vi "RW_LiveVIew.vi"(9 "Task":T2(ring), 11 "Plots":refnum<vi>[](array[refnum])) -> ()   [LabVIEW 2022 SP3]
uses:
  <vilib>/Utility/miscctls.llb/LVRangeTypeDef.ctl
panel:
  out "Data":T1[][](array[typedef])
  out "Pref Path":path
  out "File Out":string
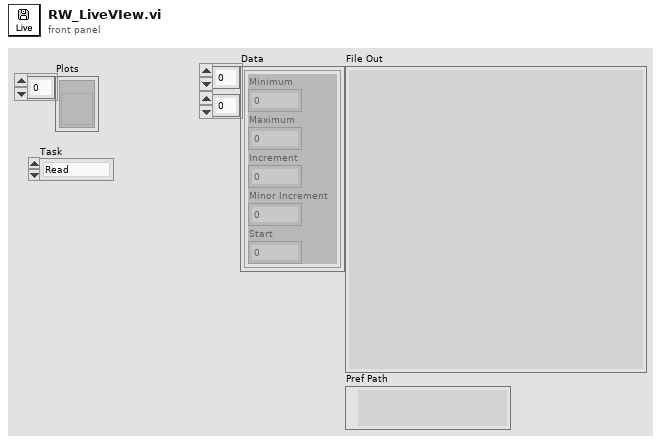
[diagram p1: front panel]
types:
  T1 = typedef "LVRangeTypeDef.ctl" = cluster{"Minimum":dbl, "Maximum":dbl, "Increment":dbl, "Minor Increment":dbl, "Start":dbl}
  T2 = enum16{"Read", "Write", "Init", "remember", "retrieve"}
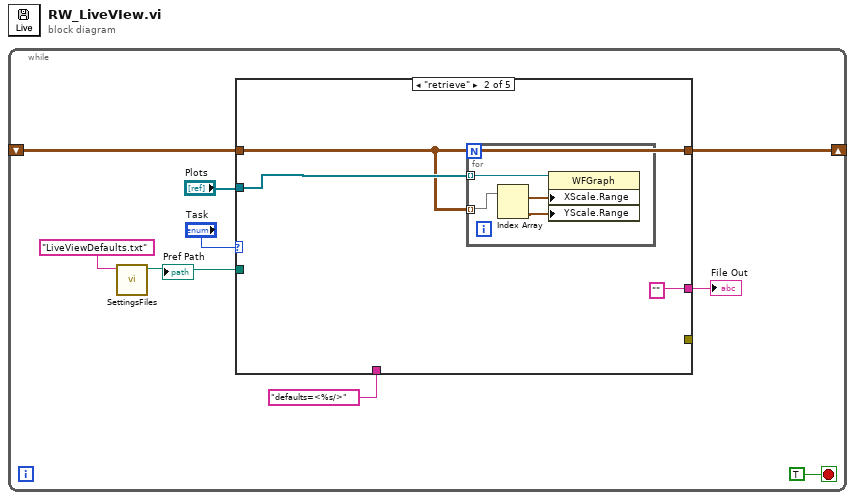
[diagram p0: block diagram]
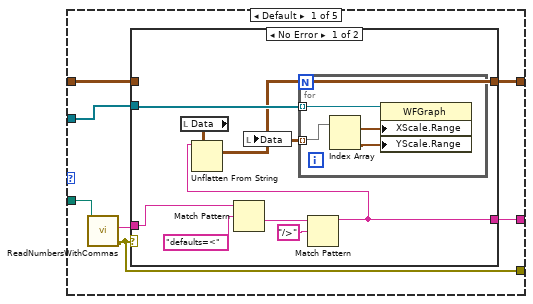
[diagram p2: hidden frame]
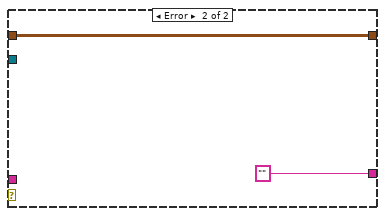
[diagram p3: hidden frame]
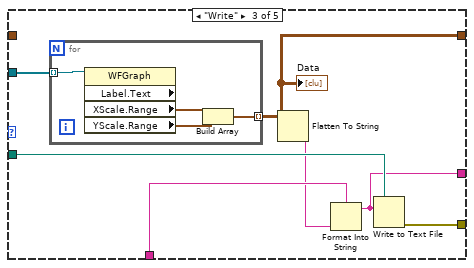
[diagram p4: hidden frame]
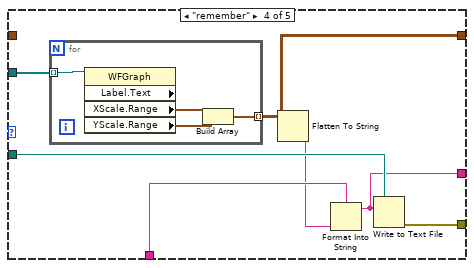
[diagram p5: hidden frame]
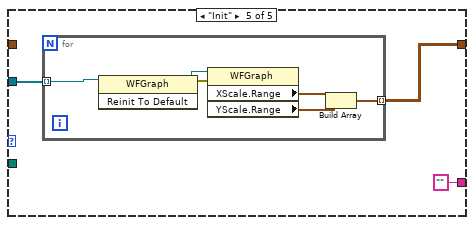
[diagram p6: hidden frame]
diagram:
  n1 = while {
    shift-right: [w3] -> _
    shift-left: _ -> [w2]
    stop <- TRUE stop-if-true
    n2 = call "SettingsFiles.vi"("settings file name"="LiveViewDefaults.txt" ("name or relative path")) -> ("file path"=w4:path)  [unwired: 9 in, 1 out]
    "Pref Path" <- w4
    n3 = case shown="\"retrieve\"" "Task" {
      tunnel: w4 -> [w16 _ w44 w55 _]
      tunnel: [w14 _ w43 w54 _] -> _
      tunnel: [w13 "" ("Notes") w39 w50 "" ("Notes")] -> w9
      tunnel: "defaults=<%s/>" ("format string") -> [_ _ w42 w53 _]
      tunnel: "Plots" -> [w12 w33 w41 w52 w62]
      tunnel: [w11 w32 w38 w49 w60] -> w3
      tunnel: w2 -> [w10 w32 _ _ _]
      frame Default {
        n4 = call "ReadNumbersWithCommas.vi"("file (use dialog)"=w16) -> ("error out"=w14:errorcluster, "text"=w15:string)  [unwired: 7 in, 2 out]
        n5 = case shown="No Error" w14 {
          tunnel: [w18 "" ("Notes")] -> w13
          tunnel: w15 -> [w24 _]
          tunnel: w12 -> [w19 _]
          tunnel: [w17 w29] -> w11
          tunnel: w10 -> [_ w29]
          frame No Error {
            n6 = local read "Data"() -> (w20:T1[][])
            n7 = Match Pattern(string=w24, regular expression="defaults=<" ("format string")) -> (after substring=w23:string)  [unwired: 1 in, 3 out]
            n8 = Match Pattern(string=w23, regular expression="/>" ("format string")) -> (before substring=w18:string)  [unwired: 1 in, 3 out]
            n9 = Unflatten From String(type=w20, binary string=w18) -> (value=w17:T1[][])  [unwired: 3 in, 2 out]
            n10 = local write "Data"(w17) -> ()
            n11 = for {
              tunnel: w19 -> [w28] mode=indexing
              tunnel: w17 -> [w27] mode=indexing
              n12 = Index Array(array=w27) -> (element #1=w26:T1, element #2=w25:T1)  [unwired: 2 in]
              n13 = property on="Property Node" class="WFGraph"(reference=w28, "XScale.Range"=w26, "YScale.Range"=w25) -> ()  [unwired: 1 in, 2 out]
            }
          }
          frame Error {
          }
        }
      }
      frame "retrieve" {
        n14 = for {
          tunnel: w33 -> [w37] mode=indexing
          tunnel: w32 -> [w36] mode=indexing
          n15 = Index Array(array=w36) -> (element #1=w35:T1, element #2=w34:T1)  [unwired: 2 in]
          n16 = property on="Property Node" class="WFGraph"(reference=w37, "XScale.Range"=w35, "YScale.Range"=w34) -> ()  [unwired: 1 in, 2 out]
        }
      }
      frame "Write" {
        n17 = for {
          tunnel: w41 -> [w48] mode=indexing
          tunnel: [w45] -> w38 mode=indexing
          n18 = property on="Property Node" class="WFGraph" props=["Label", "Text", "XScale", "Range", "YScale", "Range"](reference=w48) -> ("XScale.Range"=w47:T1, "YScale.Range"=w46:T1)  [unwired: 1 in, 3 out]
          n19 = Build Array(w47, w46) -> (w45:T1[])
        }
        "Data" <- w38
        n20 = Flatten To String(anything=w38) -> (data string=w40:string)  [unwired: 3 in, 2 out]
        n21 = Format Into String(format string=w42, w40) -> (resulting string=w39:string)  [unwired: 2 in, 1 out]
        n22 = Write to Text File(file (use dialog)=w44, text=w39) -> (error out=w43:errorcluster)  [unwired: 2 in, 2 out]
      }
      frame "remember" {
        n23 = for {
          tunnel: w52 -> [w59] mode=indexing
          tunnel: [w56] -> w49 mode=indexing
          n24 = property on="Property Node" class="WFGraph" props=["Label", "Text", "XScale", "Range", "YScale", "Range"](reference=w59) -> ("XScale.Range"=w58:T1, "YScale.Range"=w57:T1)  [unwired: 1 in, 3 out]
          n25 = Build Array(w58, w57) -> (w56:T1[])
        }
        n26 = Flatten To String(anything=w49) -> (data string=w51:string)  [unwired: 3 in, 2 out]
        n27 = Format Into String(format string=w53, w51) -> (resulting string=w50:string)  [unwired: 2 in, 1 out]
        n28 = Write to Text File(file (use dialog)=w55, text=w50) -> (error out=w54:errorcluster)  [unwired: 2 in, 2 out]
      }
      frame "Init" {
        n29 = for {
          tunnel: w62 -> [w68] mode=indexing
          tunnel: [w65] -> w60 mode=indexing
          n30 = invoke on="Invoke Node" class="WFGraph" method="Reinit To Default"(reference=w68) -> (reference out=w64:refnum<vi>, error out=w63:errorcluster)  [unwired: 2 in, 1 out]
          n31 = property on="Property Node" class="WFGraph"(reference=w64, error in=w63) -> ("XScale.Range"=w67:T1, "YScale.Range"=w66:T1)  [unwired: 2 out]
          n32 = Build Array(w67, w66) -> (w65:T1[])
        }
      }
    }
    "File Out" <- w9
  }
